vi "Read as Byte Stream.vi"(8 "error in (no error)":errorcluster, 10 "Symbol Name":string, 11 "TwinCAT ADS in":refnum<class "TwinCAT ADS.lvclass">) -> (0 "error out":errorcluster, 1 "Byte Stream out":u8[](array[numeric]), 3 "TwinCAT ADS out":refnum<class "TwinCAT ADS.lvclass">)   [LabVIEW 2018, in "TwinCAT ADS.lvclass"]
uses:
  TwinCAT ADS.lvclass
  TwinCAT ADS.lvclass/TwinCAT ADS.ctl
  TwinCAT.Ads
  Get From Symbol Map.vi
  Get From Symbol Map Daemon.vi
  Get Symbol Map.vi
  Format String.vi
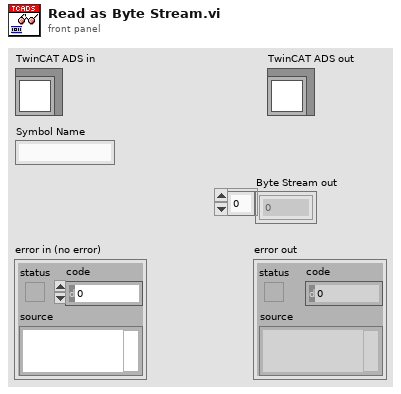
[diagram p1: front panel]
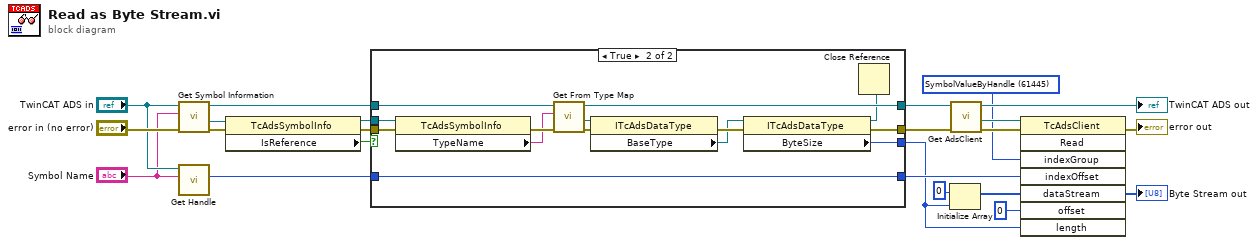
[diagram p0: block diagram]
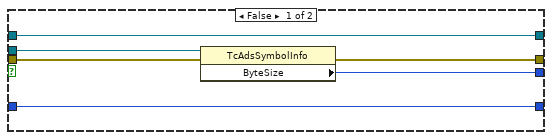
[diagram p2: hidden frame]
diagram:
  w17 = u32 61445 items=["PlcRWIB"=16384, "PlcRWOB"=16400, "PlcRWMB"=16416, "PlcRWRB"=16432, "PlcRWDB"=16448, "SymbolTable"=61440, "SymbolName"=61441, "SymbolValue"=61442, "SymbolHandleByName"=61443, "SymbolValueByName"=61444, "SymbolValueByHandle"=61445, "SymbolReleaseHandle"=61446, "SymbolInfoByName"=61447, "SymbolVersion"=61448, "SymbolInfoByNameEx"=61449, "SymbolDownload"=61450, "SymbolUpload"=61451, "SymbolUploadInfo"=61452, "SymbolNote"=61456, "IOImageRWIB"=61472, "IOImageRWIX"=61473, "IOImageRWOB"=61488, "IOImageRWOX"=61489, "IOImageClearI"=61504, "IOImageClearO"=61520, "SumCommandRead"=61568, "SumCommandWrite"=61569, "SumCommandReadWrite"=61570, "SumCommandReadEx"=61571, "SumCommandReadEx2"=61572, "SumCommandAddDevNote"=61573, "SumCommandDelDevNote"=61574, "DeviceData"=61696] ("SumCommandRead")
  n1 = call "Get Symbol Information.vi"("error in (no error)"="error in (no error)", "Symbol Name"="Symbol Name", "TwinCAT ADS in"="TwinCAT ADS in") -> ("error out"=w13:errorcluster, ".NET Symbol Information"=w12:refnum<k24>, "TwinCAT ADS out"=w11:refnum<class "TwinCAT ADS.lvclass">)  [unwired: 6 in]
  n2 = call "Get Handle.vi"("Symbol Name"="Symbol Name", "TwinCAT ADS in"="TwinCAT ADS in") -> ("Handle"=w8:i32)  [unwired: 7 in, 2 out]
  n3 = property class="TcAdsSymbolInfo"(reference=w12, error in=w13) -> (reference out=w14:refnum<k24>, error out=w15:errorcluster, "IsReference"=w16:bool)
  n4 = case shown="True" w16 {
    tunnel: w15 -> [w29 w33]
    tunnel: [w25 w41] -> w10
    tunnel: [w26 w38] -> w6
    tunnel: [w27 w36] -> w9
    tunnel: w14 -> [w28 w32]
    tunnel: w11 -> [w25 w35]
    tunnel: w8 -> [w24 w34]
    tunnel: [w24 w34] -> w7
    frame False {
      n5 = property class="TcAdsSymbolInfo"(reference=w28, error in=w29) -> (error out=w27:errorcluster, "ByteSize"=w26:i32)  [unwired: 1 out]
    }
    frame True {
      n6 = property class="TcAdsSymbolInfo"(reference=w32, error in=w33) -> (error out=w31:errorcluster, "TypeName"=w30:string)  [unwired: 1 out]
      n7 = call "Get From Type Map.vi"("error in (no error)"=w31, "Type Name"=w30, "TwinCAT ADS in"=w35) -> ("error out"=w43:errorcluster, ".NET AdsDataType"=w42:refnum<k24>, "TwinCAT ADS out"=w41:refnum<class "TwinCAT ADS.lvclass">)  [unwired: 6 in]
      n8 = property class="ITcAdsDataType"(reference=w42, error in=w43) -> (error out=w40:errorcluster, "BaseType"=w39:refnum<k24>)  [unwired: 1 out]
      n9 = property class="ITcAdsDataType"(reference=w39, error in=w40) -> (reference out=w37:refnum<k24>, error out=w36:errorcluster, "ByteSize"=w38:i32)
      n10 = Close Reference(reference=w37) -> ()  [unwired: 1 in, 1 out]
    }
  }
  n11 = Initialize Array(u8 0, w6) -> (w19:u8[])
  n12 = call "Get AdsClient.vi"("error in (no error)"=w9, "TwinCAT ADS in"=w10) -> ("error out"=w22:errorcluster, ".NET TcAdsClient"=w21:refnum<k24>, "TwinCAT ADS out"=→"TwinCAT ADS out":refnum<class "TwinCAT ADS.lvclass">)  [unwired: 7 in]
  n13 = invoke class="TcAdsClient" method="Read"(reference=w21, error in=w22, "indexGroup"=w17, "indexOffset"=w7, "dataStream"=w19, "offset"=0, "length"=w6) -> (error out=→"error out":errorcluster, "dataStream"=→"Byte Stream out":u8[])  [unwired: 1 in, 6 out]
